vi "PAM Save.vi"(0 "icListen #":i32, 1 "Path":path) -> ()   [LabVIEW 2020]
uses:
  icListen 1 Initialized.vi
  icListen 1 Serial Number.vi
  icListen 1 Position.vi
  icListen 2 Initialized.vi
  icListen 2 Serial Number.vi
  icListen 2 Position.vi
  icListen 3 Initialized.vi
  icListen 3 Serial Number.vi
  icListen 3 Position.vi
  icListen 4 Initialized.vi
  icListen 4 Serial Number.vi
  icListen 4 Position.vi
  PAM Sample Rate.vi
  PAM Volts per Bit.vi
  PAM Library.lvlib
panel:
  out "Error Out":errorcluster
  out "Queue Name":string
  out "concatenated string":string
  out "Error Out":errorcluster
  in  "Error In":errorcluster
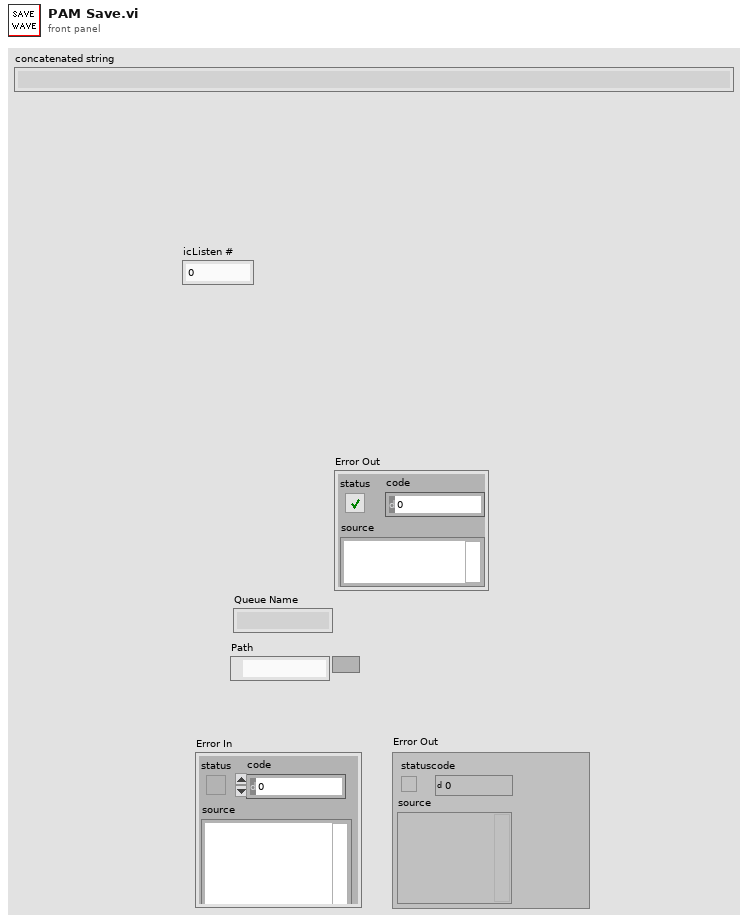
[diagram p1: front panel]
types:
  T1 = cluster{"default (0 U32) 2":i16, "default (0 U32)":i32, "unsigned 64bit integer":u64}
  T2 = cluster{"default (0 U32) 2":i16, "default (0 U32)":i32, "unsigned 64bit integer":u64}[]
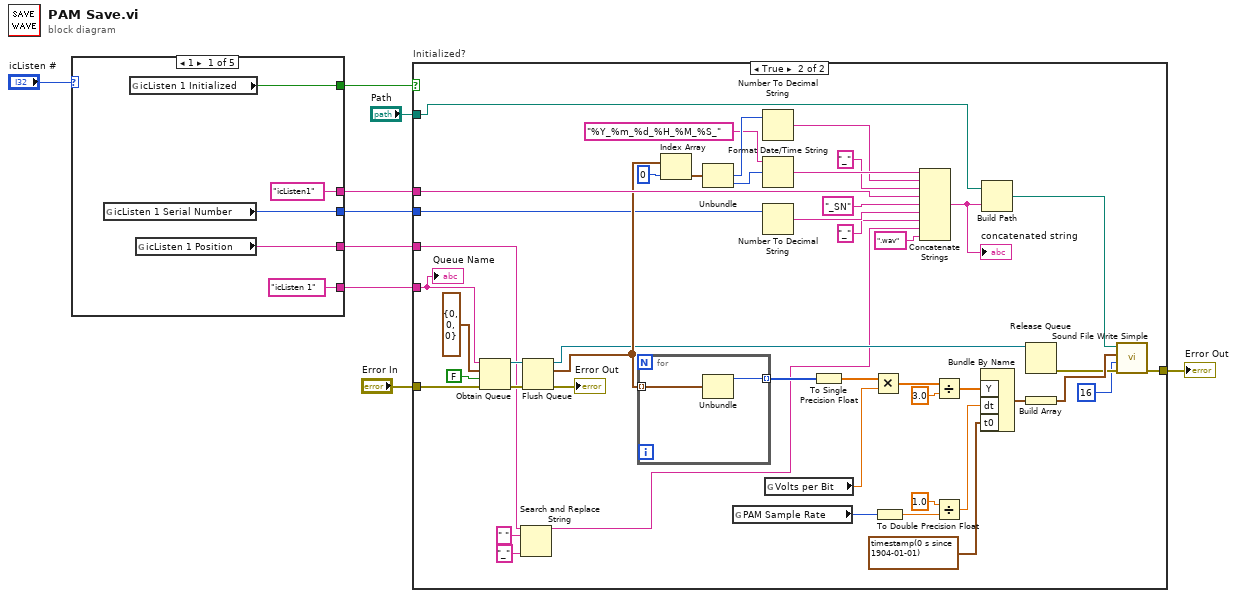
[diagram p0: block diagram]
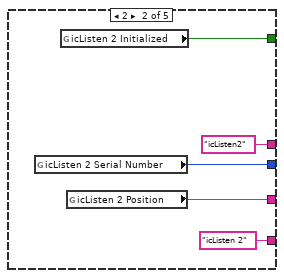
[diagram p3: hidden frame]
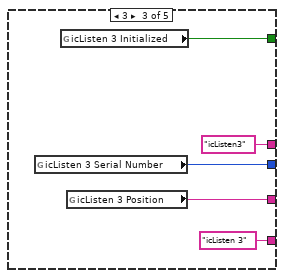
[diagram p4: hidden frame]
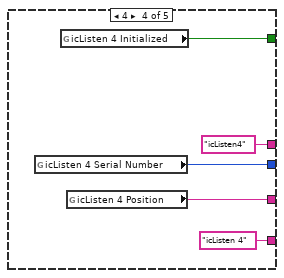
[diagram p5: hidden frame]
diagram:
  n1 = case shown="1" "icListen #" {
    tunnel: ["icListen 1" ("name (unnamed)") "icListen 2" ("File Extension") "icListen 3" ("File Extension") "icListen 4" ("File Extension") _] -> w8
    tunnel: [w14 w18 w24 w28 _] -> w6
    tunnel: ["icListen1" ("name (unnamed)") "icListen2" ("name (unnamed)") "icListen3" ("name (unnamed)") "icListen4" ("name (unnamed)") _] -> w5
    tunnel: [w11 w16 w21 w26 _] -> w2
    tunnel: [w10 w15 w20 w25 _] -> w1
    frame 1 {
      n2 = global read "icListen 1 Serial Number.vi" "icListen 1 Serial Number"() -> (w11:u16)
      n3 = global read "icListen 1 Initialized.vi" "icListen 1 Initialized"() -> (w14:bool)
      n4 = global read "icListen 1 Position.vi" "icListen 1 Position"() -> (w10:string)
    }
    frame 2 {
      n5 = global read "icListen 2 Serial Number.vi" "icListen 2 Serial Number"() -> (w16:u16)
      n6 = global read "icListen 2 Initialized.vi" "icListen 2 Initialized"() -> (w18:bool)
      n7 = global read "icListen 2 Position.vi" "icListen 2 Position"() -> (w15:string)
    }
    frame 3 {
      n8 = global read "icListen 3 Serial Number.vi" "icListen 3 Serial Number"() -> (w21:u16)
      n9 = global read "icListen 3 Initialized.vi" "icListen 3 Initialized"() -> (w24:bool)
      n10 = global read "icListen 3 Position.vi" "icListen 3 Position"() -> (w20:string)
    }
    frame 4 {
      n11 = global read "icListen 4 Serial Number.vi" "icListen 4 Serial Number"() -> (w26:u16)
      n12 = global read "icListen 4 Initialized.vi" "icListen 4 Initialized"() -> (w28:bool)
      n13 = global read "icListen 4 Position.vi" "icListen 4 Position"() -> (w25:string)
    }
    frame 5, Default {
    }
  }
  n14 = case "Initialized?" shown="True" w6 {
    tunnel: "Error In" -> [w30 w68]
    tunnel: [w30 w76] -> w9
    tunnel: w8 -> [_ w75]
    tunnel: "Path" -> [_ w69]
    tunnel: w5 -> [_ w74]
    tunnel: w2 -> [_ w38]
    tunnel: w1 -> [_ w34]
    frame False {
    }
    frame True {
      n15 = Obtain Queue(name (unnamed)=w75, element data type=T1 {"default (0 U32) 2"=0, "default (0 U32)"=0, "unsigned 64bit integer"=0} ("output cluster"), create if not found? (T)=FALSE, error in (no error)=w68) -> (queue out=w66:refnum<queue>, error out=w65:errorcluster)  [unwired: 1 in, 1 out]
      n16 = Search and Replace String(input string=w34, search string=" ", replace string="_" ("replace string (\"\")")) -> (result string=w33:string)  [unwired: 5 in, 3 out]
      n17 = Flush Queue(queue=w66, error in (no error)=w65) -> (queue out=w40:refnum<queue>, remaining elements=w42:T2, error out=→"Error Out":errorcluster)
      n18 = for {
        tunnel: w42 -> [w78] mode=indexing
        tunnel: [w77] -> w43 mode=indexing
        n19 = Unbundle(w78) -> ("default (0 U32) 2"=w77:i16)  [unwired: 2 out]
      }
      n20 = Index Array(array=w42, index=0) -> (element=w47:T1)
      n21 = Unbundle(w47) -> ("default (0 U32)"=w52:i32, "unsigned 64bit integer"=w54:u64)  [unwired: 1 out]
      n22 = global read "PAM Sample Rate.vi" "PAM Sample Rate"() -> (w67:i32)
      n23 = Number To Decimal String(number=w52) -> (decimal integer string=w50:string)  [unwired: 1 in]
      n24 = Format Date/Time String(time format string (%c)="%Y_%m_%d_%H_%M_%S_", seconds (now)=w54) -> (date/time string=w53:string)  [unwired: 1 in]
      n25 = Number To Decimal String(number=w38) -> (decimal integer string=w37:string)  [unwired: 1 in]
      n26 = global read "PAM Volts per Bit.vi" "Volts per Bit"() -> (w61:dbl)
      n27 = To Single Precision Float(number=w43) -> (single precision float=w55:sgl[])
      n28 = Multiply(x=w55, y=w61) -> (x*y=w62:dbl[])
      n29 = To Double Precision Float(number=w67) -> (double precision float=w72:dbl)
      n30 = Concatenate Strings(w53, w50, "_" ("File Extension"), w74, "_SN" ("File Extension"), w37, "_" ("string"), w33, ".wav" ("File Extension")) -> (w57:string)
      "concatenated string" <- w57
      n31 = Divide(x=w62, y=3.0) -> (x/y=w45:dbl[])
      n32 = Divide(x=1.0, y=w72) -> (x/y=w73:dbl)
      n33 = Bundle By Name("Y"=w45, "dt"=w73, "t0"=timestamp(0 s since 1904-01-01)) -> (w58:waveform(dbl))  [unwired: 1 in]
      n34 = Build Path(base path=w69, name or relative path=w57) -> (appended path=w60:path)
      n35 = Release Queue(queue=w40) -> (error out=w46:errorcluster)  [unwired: 2 in, 2 out]
      n36 = Build Array(w58) -> (w59:waveform(dbl)[])
      n37 = call <vilib>:"Sound File Write Simple.vi"("error in (no error)"=w46, "bits per sample"=16, "data"=w59, "path"=w60) -> ("error out"=w76:errorcluster)  [unwired: 6 in, 1 out]
      "Queue Name" <- w75
    }
  }
  "Error Out" <- w9
